vi "Configure Mask Test.vi"   [LabVIEW 2023, in "Keysight-DSQx3014T.lvlib"]
doc: "Configures the setttings of mast test."
uses:
  Keysight-DSQx3014T.lvlib
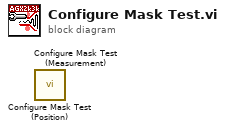
[diagram p0: block diagram]
diagram:
  n1 = call "Configure Mask Test (Position).vi"() -> ()  [unwired: 14 in, 2 out]
  n2 = call "Configure Mask Test (Measurement).vi"() -> ()  [unwired: 14 in, 2 out]
